vi "etlDynReg.vi"   [LabVIEW 2017]
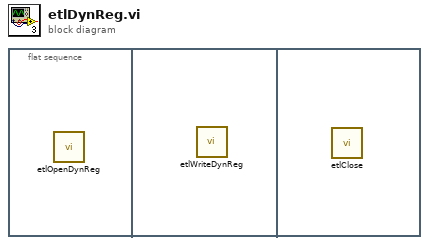
[diagram p0: block diagram]
diagram:
  n1 = flat-sequence {
    frame #0 {
      n2 = call "etlOpenDynReg.vi"() -> ()  [unwired: 12 in]
    }
    frame #1 {
      n3 = call "etlWriteDynReg.vi"() -> ()  [unwired: 12 in]
    }
    frame #2 {
      n4 = call "etlClose.vi"() -> ()  [unwired: 2 in]
    }
  }
